vi "RT Main (CVT).vi"() -> ()   [LabVIEW 2011]
uses:
  TypeDefs/Recipe Engine States.ctl
  TypeDefs/Recipe Engine Commands.ctl
  <vilib>/Platform/TimedLoop/XDataNode/timing_clust.ctl
  <vilib>/Platform/TimedLoop/XDataNode/nitl_modes.ctl
  <vilib>/Platform/TimedLoop/XDataNode/wakeup.ctl
  TypeDefs/Recipe Phase.ctl
  <vilib>/FPGAPlugInAG/cRIO-9074/niLvFpga_Open_cRIO-9074.vi
  <vilib>/rvi/interface/common/dynamic/niFpgaDynamicAddResources.vi
  <vilib>/FPGAPlugInAG/Dynamic/niLvFpga_Close_Dynamic.vi
  <vilib>/Platform/TimedLoop/XDataNode/loadnilvce.vi
  <vilib>/addons/control/pid/pid.llb/PID (DBL).vi
  <vilib>/Platform/TimedLoop/XDataNode/XDataNode.xnode
  <vilib>/rvi/interface/nirviOpenFPGA/nirviOpenFPGA.xnode
  FPGA Bitfiles/Bioreactor_FPGATarget_FPGAMain_8731874D.lvbitx
  FPGA Main.vi
  <vilib>/rvi/interface/nirviCloseFPGA/nirviCloseFPGA.xnode
  <vilib>/addons/control/pid/NI_PID_pid.lvlib
  <vilib>/Platform/TimedLoop/XDataNode/XDNodeRunTimeDep.lvlib
panel:
  out "FPGA State":enum16{"Normal Operation", "Safe State"}(ring)
  out "error out":errorcluster
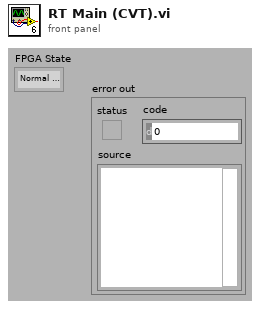
[diagram p1: front panel]
types:
  T1 = typedef "Recipe Engine Commands.ctl" = enum16{"Run Recipe", "Abort Recipe", "Exit"}
  T2 = typedef "Recipe Engine States.ctl" = enum16{"Initialize", "Wait for Cmd", "Load Phase", "Run Phase", "Exit"}
  T3 = typedef "XDNodeRunTimeDep.lvlib/timing_clust.ctl" = cluster{"Expected End [f-1]":u64, "Actual End [f-1]":u64, "Finished Late? [f-1]":bool, "Expected End [i-1]":u64, "Actual End [i-1]":u64, "Finished Late? [i-1]":bool, "Expected Start [i]":u64, "Actual Start [i]":u64, "Expected Start [f]":u64, "Actual Start [f]":u64, "Source Name":string, "Structure Name":string, "Period":i64, "Deadline":i64, "Offset":i64, "Start":i64, "Priority":i32, "Timeout":i32, "Mode":T4, "Wakeup Reason":T5, "Error":errorcluster, "Source Type":string, "Secondary Source Type":string, "Global End Time":u64, "Global Start Time":u64, "Frame Duration":u64, "Iteration Duration":u64, "Assigned CPU":i32, "I/O Scan Engine Mode":u32}
  T4 = typedef "XDNodeRunTimeDep.lvlib/nitl_modes.ctl" = enum32{"No Change", "Process missed periods, maintain original phase", "Discard missed periods, maintain original phase", "Process missed periods, ignore original phase", "Discard missed periods, ignore original phase"}
  T5 = typedef "XDNodeRunTimeDep.lvlib/wakeup.ctl" = enum32{"Normal", "Aborted", "Asynchronous wakeup", "Timing source error", "Timed loop error", "Timeout"}
  T6 = typedef "Recipe Phase.ctl" = cluster{"Temp Setpoint":dbl, "pH Setpoint":dbl, "Agitation ON":bool, "Intake ON":bool, "Waste ON":bool, "Time (s)":i32}
  T7 = cluster{"proportional gain (Kc)":dbl, "integral time (Ti, min)":dbl, "derivative time (Td, min)":dbl}
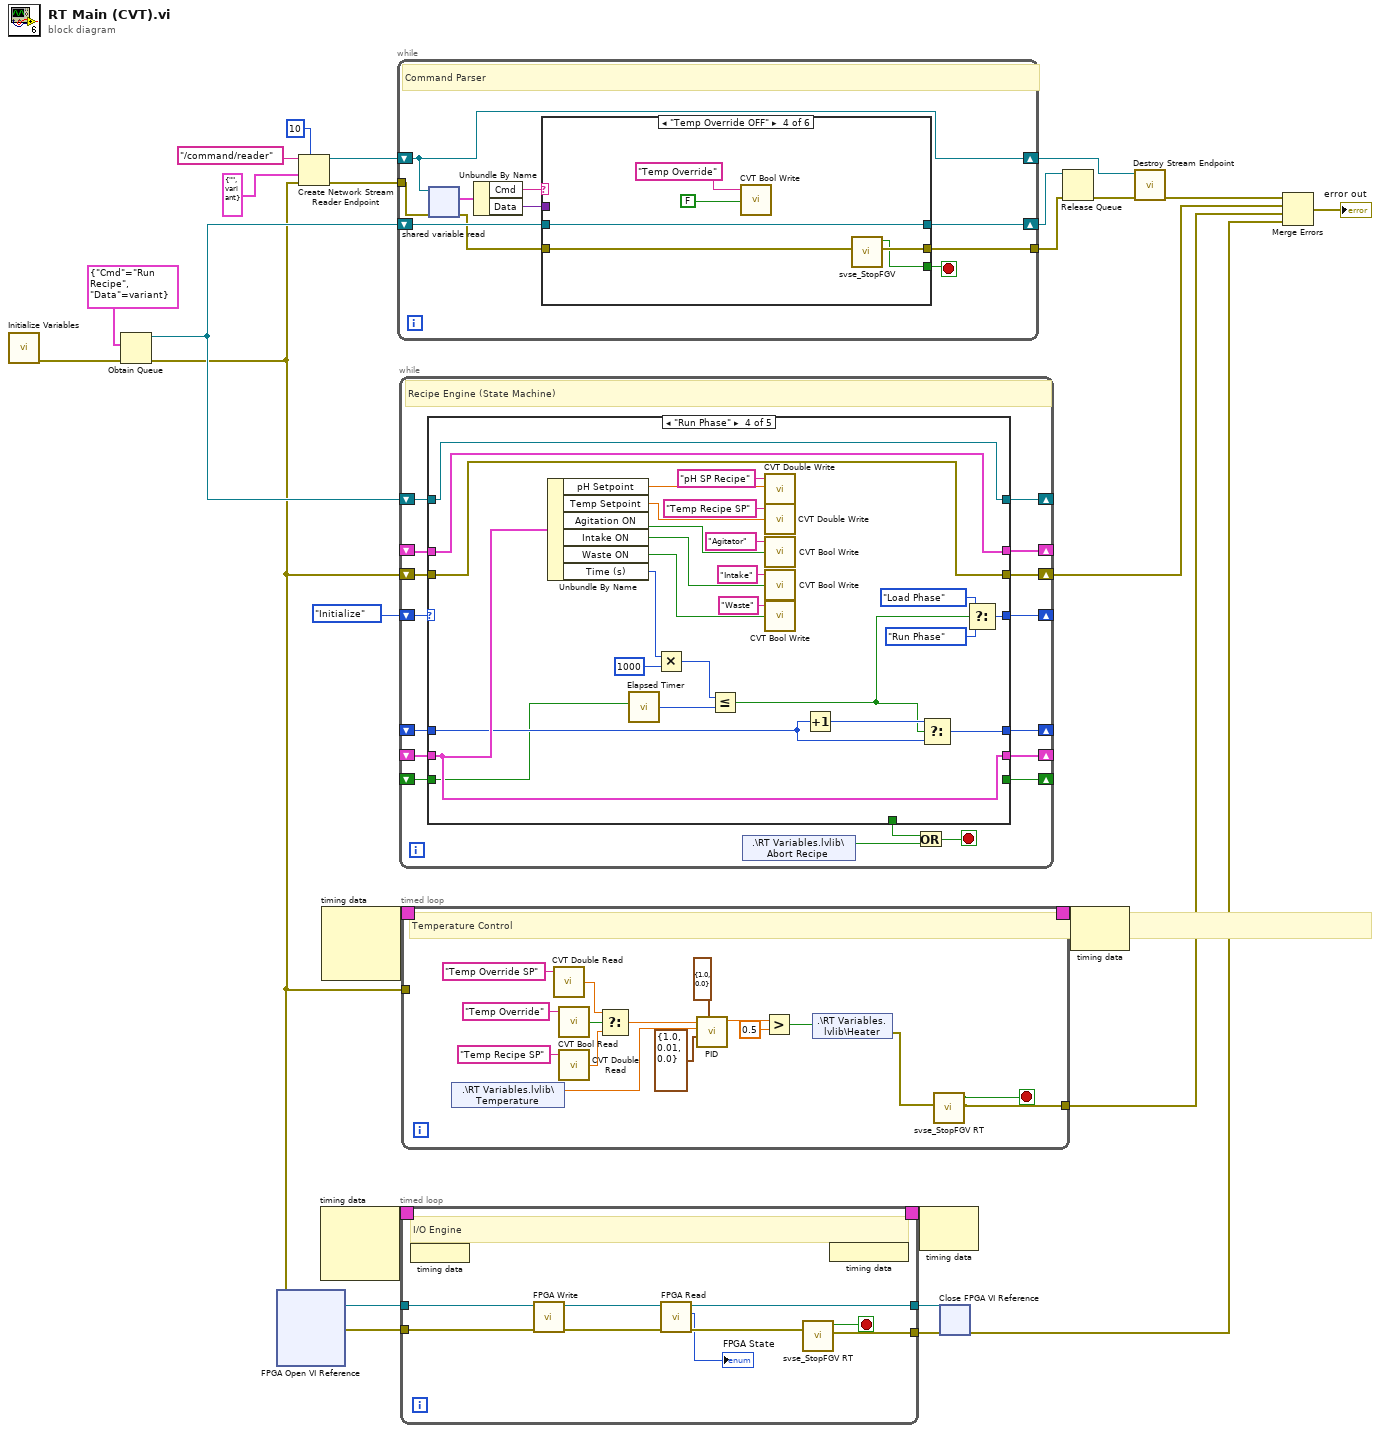
[diagram p0: block diagram]
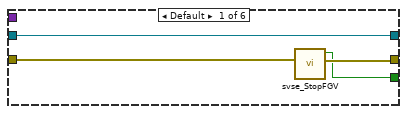
[diagram p2: hidden frame]
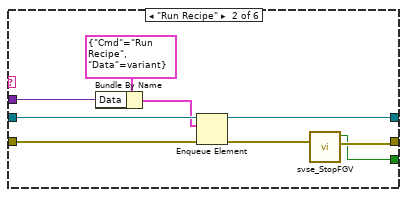
[diagram p3: hidden frame]
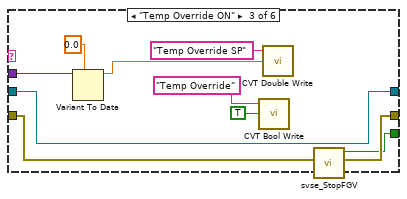
[diagram p4: hidden frame]
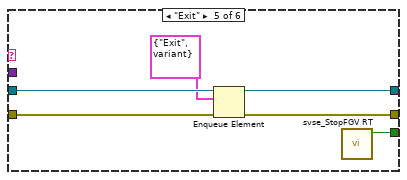
[diagram p5: hidden frame]
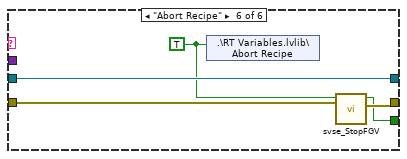
[diagram p6: hidden frame]
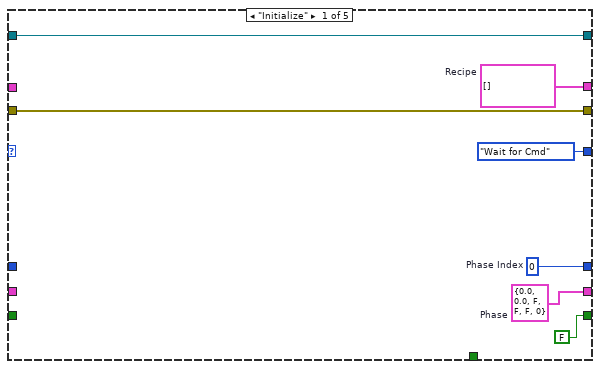
[diagram p7: hidden frame]
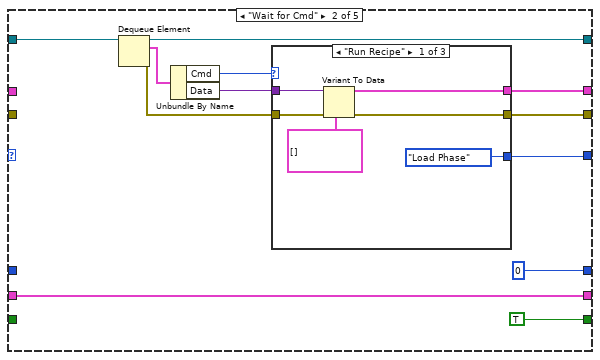
[diagram p8: hidden frame]
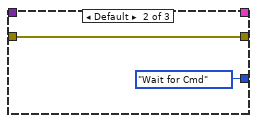
[diagram p9: hidden frame]
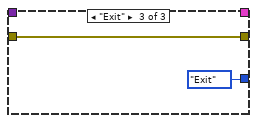
[diagram p10: hidden frame]
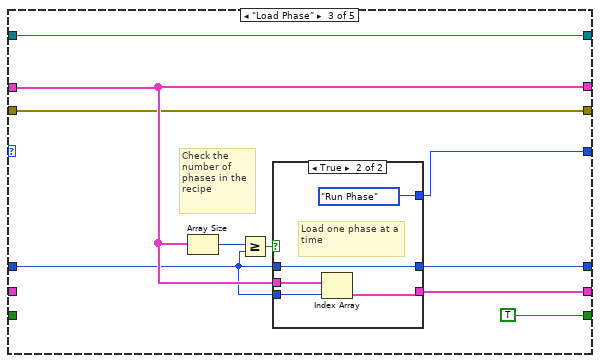
[diagram p11: hidden frame]
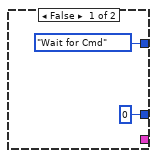
[diagram p12: hidden frame]
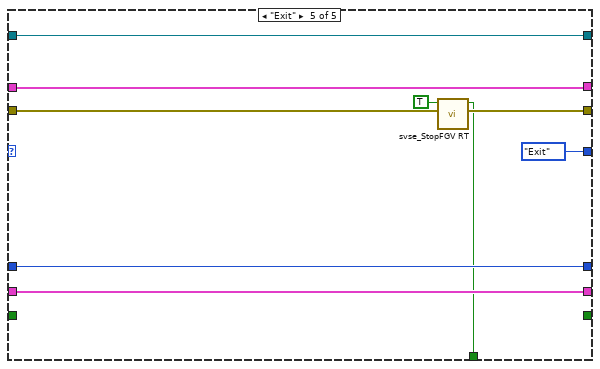
[diagram p13: hidden frame]
diagram:
  n1 = call "Initialize Variables.vi"() -> ("error out"=w20:errorcluster)  [unwired: 11 in]
  n2 = Obtain Queue(element data type=cluster{"Cmd":T1, "Data":variant} {"Cmd"=enum."Run Recipe", "Data"=variant}, error in (no error)=w20) -> (queue out=w19:refnum<queue>, error out=w2:errorcluster)  [unwired: 3 in, 1 out]
  n3 = xnode "FPGA Open VI Reference"("error in"=w2) -> ("FPGA VI Reference Out"=w6:refnum<k20>, "error out"=w5:errorcluster)  [unwired: 1 in]
  n4 = Create Network Stream Reader Endpoint(7:10 ("reader buffer size"), 8:w2, 9:cluster{"Cmd":string, "Data":variant} {"Cmd"="", "Data"=variant}, 11:"/command/reader" ("reader url")) -> (0:w21:errorcluster, 3:w23:refnum<k21>)  [unwired: 2 in]
  n5 = node-c288() -> (w8:T3)  [unwired: 3 in]
  n6 = node-c288() -> (w18:T3)  [unwired: 3 in]
  n7 = while {
    shift-right: [w33] -> w9
    shift-left: w23 -> [w33]
    shift-right: [w32] -> w16
    shift-left: w19 -> [w34]
    tunnel: w21 -> [w31]
    tunnel: [w29] -> w15
    stop <- w28 stop-if-true
    # "Command Parser"
    n8 = shared-variable-read(w33, w31) -> (w30:errorcluster, w37:cluster{"Cmd":string, "Data":variant})  [unwired: 1 in, 2 out]
    n9 = Unbundle By Name(w37) -> ("Cmd"=w36:string, "Data"=w35:variant)
    n10 = case shown="\"Temp Override OFF\"" w36 {
      tunnel: w35 -> [_ w48 w60 _ _ _]
      tunnel: w34 -> [w41 w50 w58 w66 w72 w77]
      tunnel: [w41 w46 w58 w66 w70 w77] -> w32
      tunnel: w30 -> [w40 w45 w57 w65 w71 w76]
      tunnel: [w39 w43 w56 w64 w68 w75] -> w29
      tunnel: [w38 w42 w55 w63 w67 w73] -> w28
      frame Default {
        n11 = call "svse_StopFGV.vi"("error in"=w40) -> ("error out"=w39:errorcluster, "Stop?"=w38:bool)  [unwired: 9 in]
      }
      frame "Run Recipe" {
        n12 = Bundle By Name(cluster=cluster{"Cmd":T1, "Data":variant} {"Cmd"=enum."Run Recipe", "Data"=variant}, "Data"=w48) -> (w47:cluster{"Cmd":T1, "Data":variant})
        n13 = Enqueue Element(queue=w50, element=w47, error in (no error)=w45) -> (queue out=w46:refnum<queue>, error out=w44:errorcluster)  [unwired: 1 in, 1 out]
        n14 = call "svse_StopFGV.vi"("error in"=w44) -> ("error out"=w43:errorcluster, "Stop?"=w42:bool)  [unwired: 9 in]
      }
      frame "Temp Override ON" {
        n15 = Variant To Data(type=0.0, Variant=w60) -> (data=w52:dbl)  [unwired: 1 in, 1 out]
        n16 = call <userlib>:"CVT Bool Write.vi"("Value"=TRUE ("Temp Override"), "Tag Name"="Temp Override") -> ()  [unwired: 3 in, 1 out]
        n17 = call <userlib>:"CVT Double Write.vi"("Value"=w52, "Tag Name"="Temp Override SP") -> ()  [unwired: 3 in, 1 out]
        n18 = call "svse_StopFGV.vi"("error in"=w57) -> ("error out"=w56:errorcluster, "Stop?"=w55:bool)  [unwired: 9 in]
      }
      frame "Temp Override OFF" {
        n19 = call <userlib>:"CVT Bool Write.vi"("Value"=FALSE ("Temp Override"), "Tag Name"="Temp Override") -> ()  [unwired: 3 in, 1 out]
        n20 = call "svse_StopFGV.vi"("error in"=w65) -> ("error out"=w64:errorcluster, "Stop?"=w63:bool)  [unwired: 9 in]
      }
      frame "Exit" {
        n21 = Enqueue Element(queue=w72, element=cluster{"Cmd":T1, "Data":variant} {"Cmd"=enum."Exit", "Data"=variant}, error in (no error)=w71) -> (queue out=w70:refnum<queue>, error out=w68:errorcluster)  [unwired: 1 in, 1 out]
        n22 = call "svse_StopFGV RT.vi"() -> ("Stop?"=w67:bool)  [unwired: 10 in, 1 out]
      }
      frame "Abort Recipe" {
        w74 = TRUE ("Abort")
        n23 = shared-variable ".\\RT Variables.lvlib\\Abort Recipe"(w74) -> ()  [unwired: 1 in, 1 out]
        n24 = call "svse_StopFGV.vi"("error in"=w76, "User stop? (F)"=w74) -> ("error out"=w75:errorcluster, "Stop?"=w73:bool)  [unwired: 8 in]
      }
    }
  }
  n25 = while "Recipe" {
    shift-right: [w92] -> _
    shift-left: w19 -> [w93]
    shift-right: [w91] -> _
    shift-left: _ -> [w89]
    shift-right: [w90] -> _
    shift-left: Recipe_Engine_States."Initialize" ("Enum") -> [w94]
    shift-right: [w87] -> _
    shift-left: _ -> [w88]
    shift-right: [w86] -> _
    shift-left: _ -> [w85]
    shift-right: [w83] -> _
    shift-left: _ -> [w82]
    shift-right: [w80] -> w14
    shift-left: w2 -> [w79]
    stop <- w84 stop-if-true
    # "Recipe Engine (State Machine)"
    n26 = case shown="\"Run Phase\"" w94 {
      tunnel: w93 -> [w95 w113 w133 w162 w175]
      tunnel: [w95 w112 w133 w162 w175] -> w92
      tunnel: [w101 w108 w131 w161 w174] -> w91
      tunnel: [Recipe_Engine_States."Wait for Cmd" ("Enum") w107 w128 w163 Recipe_Engine_States."Exit" ("Enum")] -> w90
      tunnel: w89 -> [_ _ w131 w161 w174]
      tunnel: w88 -> [_ _ w127 w164 w172]
      tunnel: [w99 0 ("Current Phase") w126 w165 w172] -> w87
      tunnel: [w100 w105 w130 w166 w171] -> w86
      tunnel: w85 -> [_ w105 _ w166 w171]
      tunnel: [FALSE TRUE TRUE _ _] -> w83
      tunnel: w82 -> [_ _ _ w160 _]
      tunnel: [w96 w102 w124 w159 w169] -> w80
      tunnel: w79 -> [w96 _ w124 w159 w170]
      tunnel: [_ _ _ _ w168] -> w78
      frame "Initialize" {
        w99 = 0  # Phase Index
        w100 = T6 {"Temp Setpoint"=0.0, "pH Setpoint"=0.0, "Agitation ON"=FALSE, "Intake ON"=FALSE, "Waste ON"=FALSE, "Time (s)"=0}  # Phase
        w101 = T6[] []  # Recipe
      }
      frame "Wait for Cmd" {
        n27 = Dequeue Element(queue=w113) -> (queue out=w112:refnum<queue>, element=w111:cluster{"Cmd":T1, "Data":variant}, error out=w103:errorcluster)  [unwired: 2 in, 1 out]
        n28 = Unbundle By Name(w111) -> ("Cmd"=w110:T1, "Data"=w109:variant)
        n29 = case shown="\"Run Recipe\"" w110 {
          tunnel: w109 -> [w119 _ _]
          tunnel: [w117 _ _] -> w108
          tunnel: [Recipe_Engine_States."Load Phase" ("Enum") Recipe_Engine_States."Wait for Cmd" ("Enum") Recipe_Engine_States."Exit" ("Enum")] -> w107
          tunnel: w103 -> [w115 w120 w122]
          tunnel: [w114 w120 w122] -> w102
          frame "Run Recipe" {
            n30 = Variant To Data(error in=w115, type=T6[] [], Variant=w119) -> (data=w117:T6[], error out=w114:errorcluster)
          }
          frame Default {
          }
          frame "Exit" {
          }
        }
      }
      frame "Load Phase" {
        # "Check the number of phases in the recipe"
        n31 = Array Size(array=w131) -> (size(s)=w132:i32)
        n32 = Greater Or Equal?(x=w132, y=w127) -> (x >= y?=w129:bool)
        n33 = case shown="True" w129 {
          tunnel: w131 -> [_ w140]
          tunnel: [_ w139] -> w130
          tunnel: w127 -> [_ w138]
          tunnel: [Recipe_Engine_States."Wait for Cmd" ("Enum") Recipe_Engine_States."Run Phase" ("Enum")] -> w128
          tunnel: w127 -> [_ w136]
          tunnel: [0 ("Current Phase") w136] -> w126
          frame False {
          }
          frame True {
            # "Load one phase at a time"
            n34 = Index Array "Index Array"(array=w140, index=w138) -> (element=w139:T6)
          }
        }
      }
      frame "Run Phase" {
        n35 = Unbundle By Name(w166) -> ("pH Setpoint"=w144:dbl, "Temp Setpoint"=w142:dbl, "Agitation ON"=w147:bool, "Intake ON"=w146:bool, "Waste ON"=w145:bool, "Time (s)"=w154:i32)
        n36 = call "Elapsed Timer.vi"("Reset Timer"=w160) -> ("Elapsed Time (ms)"=w151:u32)  [unwired: 10 in]
        n37 = Multiply(x=w154, y=1000) -> (x*y=w152:i32)
        n38 = Less Or Equal?(x=w152, y=w151) -> (x <= y?=w155:bool)
        n39 = call <userlib>:"CVT Double Write.vi"("Value"=w144, "Tag Name"="pH SP Recipe") -> ()  [unwired: 3 in, 1 out]
        n40 = call <userlib>:"CVT Double Write.vi"("Value"=w142, "Tag Name"="Temp Recipe SP") -> ()  [unwired: 3 in, 1 out]
        n41 = call <userlib>:"CVT Bool Write.vi"("Value"=w147, "Tag Name"="Agitator") -> ()  [unwired: 3 in, 1 out]
        n42 = call <userlib>:"CVT Bool Write.vi"("Value"=w146, "Tag Name"="Intake") -> ()  [unwired: 3 in, 1 out]
        n43 = call <userlib>:"CVT Bool Write.vi"("Value"=w145, "Tag Name"="Waste") -> ()  [unwired: 3 in, 1 out]
        n44 = Increment(x=w164) -> (x+1=w158:i32)
        n45 = Select(t=w158, s=w155, f=w164) -> (s? t:f=w165:i32)
        n46 = Select(t=Recipe_Engine_States."Load Phase" ("Enum"), s=w155, f=Recipe_Engine_States."Run Phase" ("Enum")) -> (s? t:f=w163:T2)
      }
      frame "Exit" {
        n47 = call "svse_StopFGV RT.vi"("error in"=w170, "User stop? (F)"=TRUE) -> ("error out"=w169:errorcluster, "Stop?"=w168:bool)  [unwired: 8 in]
      }
    }
    n48 = shared-variable ".\\RT Variables.lvlib\\Abort Recipe"() -> (w81:bool)  [unwired: 1 in, 1 out]
    n49 = Or(x=w78, y=w81) -> (x .or. y?=w84:bool)
  }
  n50 = timed-loop "I/O Engine" {
    timing: w8 -> [_]
    timing-out: [_] -> w7
    tunnel: w6 -> [w184]
    tunnel: w5 -> [w183]
    tunnel: [w181] -> w4
    tunnel: [w177] -> w1
    stop <- w180 stop-if-true
    # "I/O Engine"
    n51 = node-c288() -> ()  [unwired: 1 in]
    n52 = call "FPGA Write.vi"("error in"=w183, "Refnum in"=w184) -> ("error out"=w178:errorcluster, "Refnum out"=w179:refnum<k20>)  [unwired: 8 in]
    n53 = call "FPGA Read.vi"("error in (no error)"=w178, "Refnum in"=w179) -> ("error out"=w182:errorcluster, "FPGA State"=→"FPGA State":enum16{"Normal Operation", "Safe State"}, "FPGA VI Reference Out"=w177:refnum<k20>)  [unwired: 6 in]
    n54 = call "svse_StopFGV RT.vi"("error in"=w182) -> ("error out"=w181:errorcluster, "Stop?"=w180:bool)  [unwired: 9 in]
    n55 = node-c288() -> ()  [unwired: 1 out]
  }
  n56 = timed-loop "Temp Ctrl" {
    timing: w18 -> [_]
    timing-out: [_] -> w17
    tunnel: w2 -> [_]
    tunnel: [w195] -> w12
    stop <- w194 stop-if-true
    # "Temperature Control"
    n57 = shared-variable ".\\RT Variables.lvlib\\Temperature"() -> (w197:dbl)  [unwired: 1 in, 1 out]
    n58 = call <userlib>:"CVT Double Read.vi"("Tag Name"="Temp Override SP") -> ("Value"=w187:dbl)  [unwired: 3 in, 1 out]
    n59 = call <userlib>:"CVT Bool Read.vi"("Tag Name"="Temp Override") -> ("Value"=w190:bool)  [unwired: 3 in, 1 out]
    n60 = call <userlib>:"CVT Double Read.vi"("Tag Name"="Temp Recipe SP") -> ("Value"=w191:dbl)  [unwired: 3 in, 1 out]
    n61 = Select(t=w187, s=w190, f=w191) -> (s? t:f=w202:dbl)
    n62 = call-poly <vilib>:"PID.vi"("output range"=cluster{"output high":dbl, "output low":dbl} {"output high"=1.0, "output low"=0.0}, "PID gains"=T7 {"proportional gain (Kc)"=1.0, "integral time (Ti, min)"=0.01, "derivative time (Td, min)"=0.0}, "process variable"=w197, "setpoint"=w202) -> ("output"=w199:dbl)  [unwired: 6 in, 1 out]
    n63 = Greater?(x=w199, y=0.5) -> (0:w196:bool)
    n64 = shared-variable ".\\RT Variables.lvlib\\Heater"(w196) -> (error out=w193:errorcluster)  [unwired: 1 in]
    n65 = call "svse_StopFGV RT.vi"("error in"=w193) -> ("error out"=w195:errorcluster, "Stop?"=w194:bool)  [unwired: 9 in]
  }
  n66 = node-c288(w7) -> ()  [unwired: 1 out]
  n67 = xnode "Close FPGA VI Reference"("FPGA VI Reference In"=w1, "error in"=w4) -> ("error out"=w3:errorcluster)
  n68 = Release Queue(queue=w16, error in (no error)=w15) -> (error out=w11:errorcluster)  [unwired: 1 in, 2 out]
  n69 = node-c288(w17) -> ()  [unwired: 1 out]
  n70 = call "Destroy Stream Endpoint.vi"("error in (no error)"=w11, "Refnum in"=w9) -> ("error out"=w10:errorcluster)  [unwired: 9 in]
  n71 = Merge Errors(w10, w14, w12, w3) -> (→"error out":errorcluster)
